vi "PID function.vi"(6 "D":dbl, 8 "I":dbl, 9 "P":dbl, 10 "Current Field":dbl[unit], 11 "Field Desired":dbl[unit]) -> (1 "Deriv":dynamicdata(waveform), 2 "Integral":dynamicdata(waveform), 3 "Numeric":dbl)   [LabVIEW 2009, in "Varian.lvlib"]
uses:
  Varian.lvlib
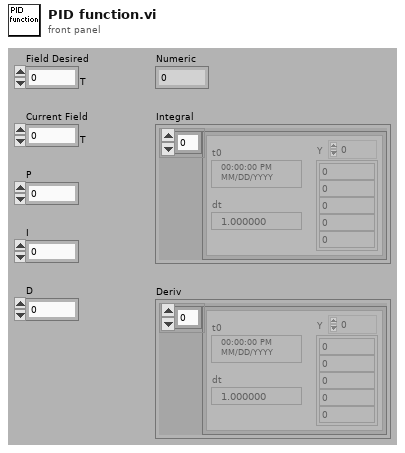
[diagram p1: front panel]
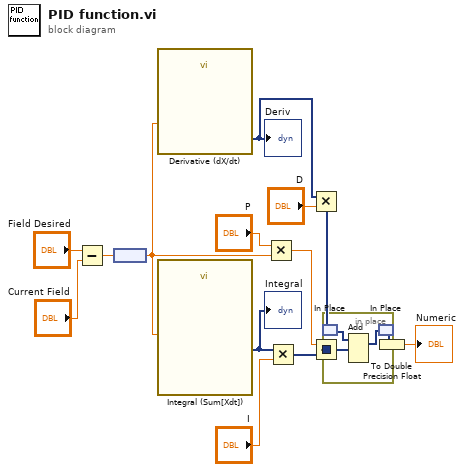
[diagram p0: block diagram]
diagram:
  n1 = Subtract(x="Field Desired", y="Current Field") -> (x-y=w9:dbl[unit])
  n2 = node(w9) -> (w1:dbl)
  n3 = call "Derivative (dX/dt)"("Signals"=w1) -> ("Result"=w15:dynamicdata)  [unwired: 1 in, 5 out]
  "Deriv" <- w15
  n4 = call "Integral (Sum[Xdt])"("Signals"=w1) -> ("Result"=w14:dynamicdata)  [unwired: 1 in, 5 out]
  "Integral" <- w14
  n5 = Multiply(x="P", y=w1) -> (x*y=w5:dbl)
  n6 = Multiply(x=w14, y="I") -> (x*y=w6:dynamicdata)
  n7 = Multiply(x=w15, y="D") -> (x*y=w8:dynamicdata)
  n8 = Add(x=w5, y=w6) -> (x+y=w7:dynamicdata)
  n9 = in-place {
    in-place-border: w7 -> [w16]
    n10 = in-place-match #1(w8) -> (w17:dynamicdata)
    n11 = Add(1:w16, 2:w17) -> (0:w18:dynamicdata)  [unwired: 1 in, 1 out]
    n12 = in-place-match #1(w18) -> (w10:dynamicdata)
  }
  n13 = To Double Precision Float(number=w10) -> (double precision float=→"Numeric":dbl)
